vi "Write OPCUA.lvclass.vi"(8 "error in (no error)":errorcluster, 10 "OPCUA.lvlib:OPCUA.lvclass":refnum<class "OPCUA.lvclass">, 11 "Model_AMC in":refnum<class "Model_AMC.lvclass">) -> (0 "error out":errorcluster, 3 "Model_AMC out":refnum<class "Model_AMC.lvclass">)   [LabVIEW 2021, in "Model_AMC.lvclass"]
uses:
  Model_AMC.lvclass
  Model_AMC.lvclass/Model_AMC.ctl
  <userlib>/John_Lib/OPCUA/OPCUA.lvclass
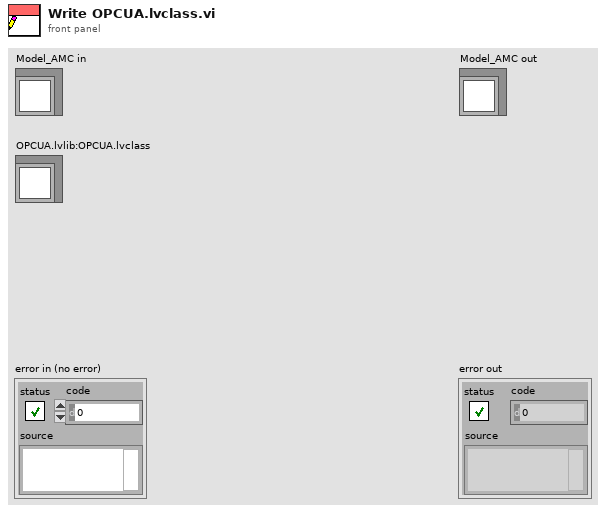
[diagram p1: front panel]
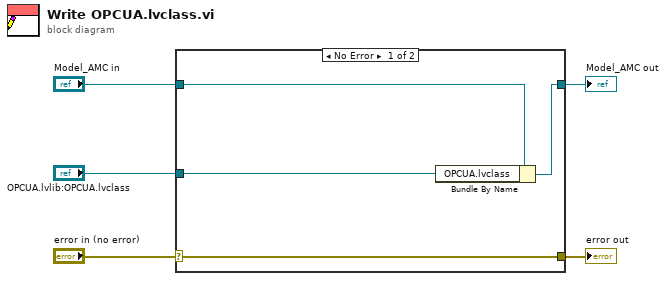
[diagram p0: block diagram]
diagram:
  n1 = case shown="No Error" "error in (no error)" {
    selector: "error in (no error)" -> [w9 w10]
    tunnel: [w9 w10] -> w4
    tunnel: [w7 w11] -> w2
    tunnel: "Model_AMC in" -> [w8 w11]
    tunnel: "OPCUA.lvlib:OPCUA.lvclass" -> [w6 _]
    frame No Error {
      n2 = Bundle By Name(cluster=w8, "OPCUA.lvclass"=w6) -> (w7:refnum<class "Model_AMC.lvclass">)
    }
    frame Error {
    }
  }
  "error out" <- w4
  "Model_AMC out" <- w2
